vi "Query Heat Alarm.vi"(8 "error in (no error)":errorcluster, 11 "MC switch refnum in":refnum<k24>) -> (0 "error out":errorcluster, 2 "exceeds specified limit?":bool, 3 "MC switch refnum out":refnum<k24>)   [LabVIEW 2019, in "Minicircuit RF Switch Box.lvlib"]
doc: "Query the alarm notification if any of the internal temperature sensors exceeds the factory programmed limits (45°C on the PCB or 48°C on the internal switch case)."
uses:
  <instrlib>/LV_Minicircuit_RF_Switch/Minicircuit RF Switch Box.lvlib
  C:/Program Files (x86)/National Instruments/LabVIEW 2019/instr.lib/LV_Minicircuit_RF_Switch/mcl_RF_Switch_Controller_NET45.dll
  mcl_RF_Switch_Controller_NET45.dll
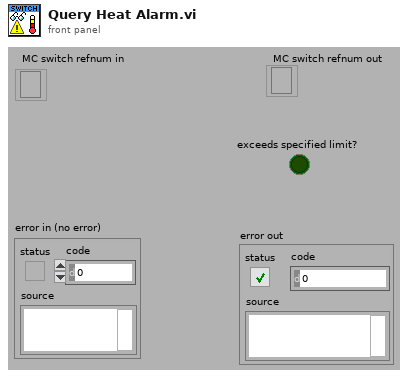
[diagram p1: front panel]
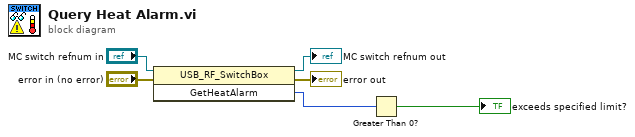
[diagram p0: block diagram]
diagram:
  n1 = invoke class="USB_RF_SwitchBox" method="GetHeatAlarm"(reference="MC switch refnum in", error in="error in (no error)") -> (reference out=→"MC switch refnum out":refnum<k24>, error out=→"error out":errorcluster, "GetHeatAlarm"=w2:i32)  [unwired: 1 in]
  n2 = Greater Than 0?(x=w2) -> (x > 0?=→"exceeds specified limit?":bool)
